vi "Pulse.vi"(8 "error in (no error)":errorcluster, 9 "Sender":string, 10 "Pulse In":enum16{"Low", "High"}(ring), 11 "Conjunction In":refnum<class "Conjunction.lvclass">) -> (0 "error out":errorcluster, 1 "Receivers":string[](array[string]), 2 "Pulse Out":enum16{"Low", "High"}(ring), 3 "Conjunction Out":refnum<class "Conjunction.lvclass">)   [LabVIEW 2021, in "Conjunction.lvclass"]
uses:
  Conjunction.lvclass
  Conjunction.lvclass/Conjunction.ctl
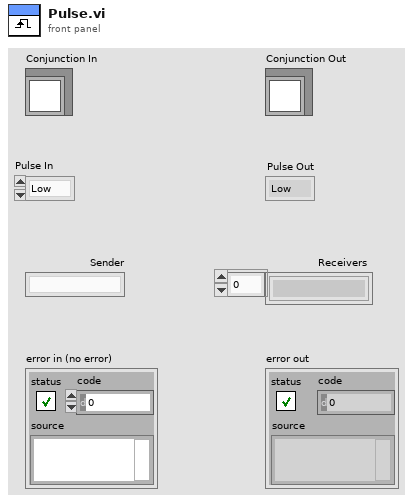
[diagram p1: front panel]
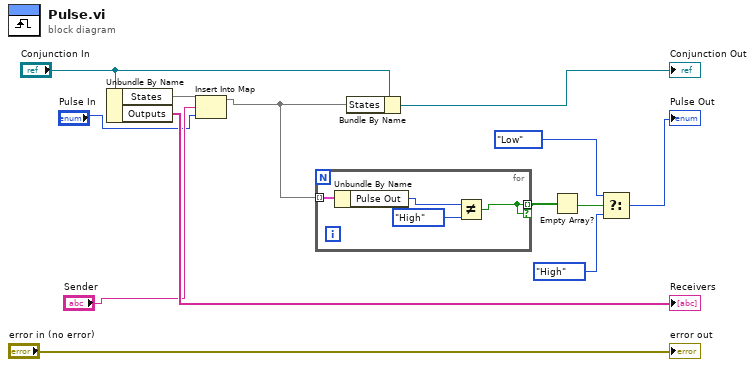
[diagram p0: block diagram]
diagram:
  n1 = Unbundle By Name("Conjunction In") -> ("States"=w11:map{string, enum16{"Low", "High"}}, "Outputs"=→"Receivers":string[])
  n2 = Insert Into Map(map in=w11, key="Sender", value="Pulse In") -> (map out=w6:map{string, enum16{"Low", "High"}})  [unwired: 2 out]
  n3 = for {
    tunnel: w6 -> [w17] mode=indexing
    tunnel: [w15] -> w5 mode=indexing if=w15
    n4 = Unbundle By Name(w17) -> ("Pulse Out"=w16:enum16{"Low", "High"})
    n5 = Not Equal?(x=w16, y=enum16{"Low", "High"}."High") -> (x != y?=w15:bool)
  }
  n6 = Bundle By Name(cluster="Conjunction In", "States"=w6) -> (→"Conjunction Out":refnum<class "Conjunction.lvclass">)
  n7 = Empty Array?(array=w5) -> (empty?=w4:bool)
  n8 = Select(t=enum16{"Low", "High"}."Low" ("y"), s=w4, f=enum16{"Low", "High"}."High" ("y")) -> (s? t:f=→"Pulse Out":enum16{"Low", "High"})
  "error out" <- "error in (no error)"
